vi "test RT Config - Dual RT Sweep.vi"(8 "error in (no error)":errorcluster, 11 "RT Config in":refnum<class "RT Config.lvclass">) -> (0 "error out":errorcluster, 3 "RT Config out":refnum<class "RT Config.lvclass">)   [LabVIEW 2016, in "RT Config.lvclass"]
uses:
  RT Config.lvclass
  Remote Terminal/TypeDefs/RT Configuration.ctl
  Remote Terminal/Remote Terminal.lvclass
  1553 Board/1553 Board.lvclass
  1553 Component/1553 Component.lvclass
  1553 SubComponent/TypeDefs/Scaling Information.ctl
  1553 SubComponent/1553 SubComponent.lvclass
  1553 SubComponent/TypeDefs/Parameter Table Data.ctl
  Remote Terminal/TypeDefs/Command Type.ctl
  Remote Terminal/TypeDefs/Command Configuration.ctl
  D:/SVN/Products/BCI-1553/Software/Development/2016/RealTime/1553 SubComponent/1553 SubComponent.lvclass
  PPLs/FPGA Interface.lvlibp/FPGA Interface/FPGA Interface.lvclass
  Utilities/FPGA Interface/FPGA Interface.lvclass
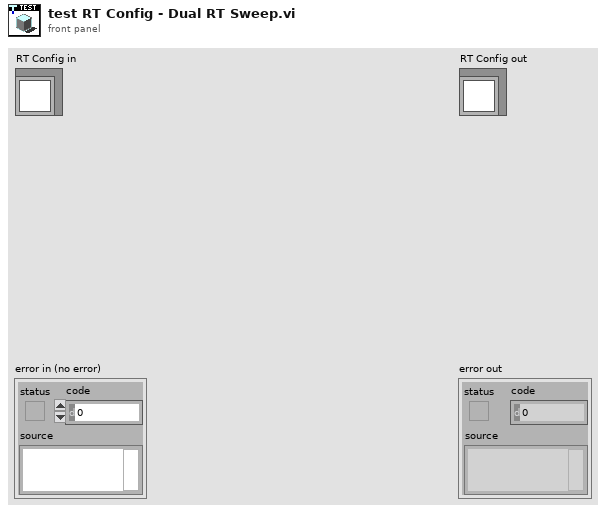
[diagram p1: front panel]
types:
  T1 = typedef "BCI-1553 API.lvlib/Remote Terminal.lvclass/RT Configuration.ctl" = cluster{"RT-RT TimeOut (us)":u8, "Inhibit Bus A":bool, "Inhibit Bus B":bool, "Broadcast CMD Invalid":bool, "UnDef MCs Invalid":bool, "Notice 2 Data Storage":bool, "SMCP":bool, "Temp RX Buffer":bool, "Alt BIT Enable":bool, "Auto Bus Shutdown":bool, "MC 17 Sync":u8, "MC 16 SR Reset":bool, "MC 8 Reset":bool}
  T2 = typedef "BCI-1553 API.lvlib/Remote Terminal.lvclass/Command Type.ctl" = enum16{"Transmit", "Receive", "Mode Code Tx", "Mode Code Rx"}
  T3 = typedef "BCI-1553 API.lvlib/Remote Terminal.lvclass/Command Configuration.ctl" = cluster{"Command Type":T2, "Mode Code ID (1-32)":u16, "SubAddress (1-30)":u16, "Word Count (1-32)":u16, "Illegal Command":bool, "Broadcast":bool, "Data":u16[], "Data Fields":T4[]}
  T4 = typedef "BCI-1553 API.lvlib/1553 SubComponent.lvclass/Parameter Table Data.ctl" = cluster{"Parameter Name":string, "Base Word":u16, "Address":u16, "Value":u64, "Mask":u16[], "Scaling Info":T5}
  T5 = typedef "BCI-1553 API.lvlib/1553 SubComponent.lvclass/Scaling Information.ctl" = cluster{"Bit Offset":i32, "Bit Count":i32, "LSB Resolution":dbl, "2's Complement":bool, "Big Endian":bool, "Sign Bit":bool}
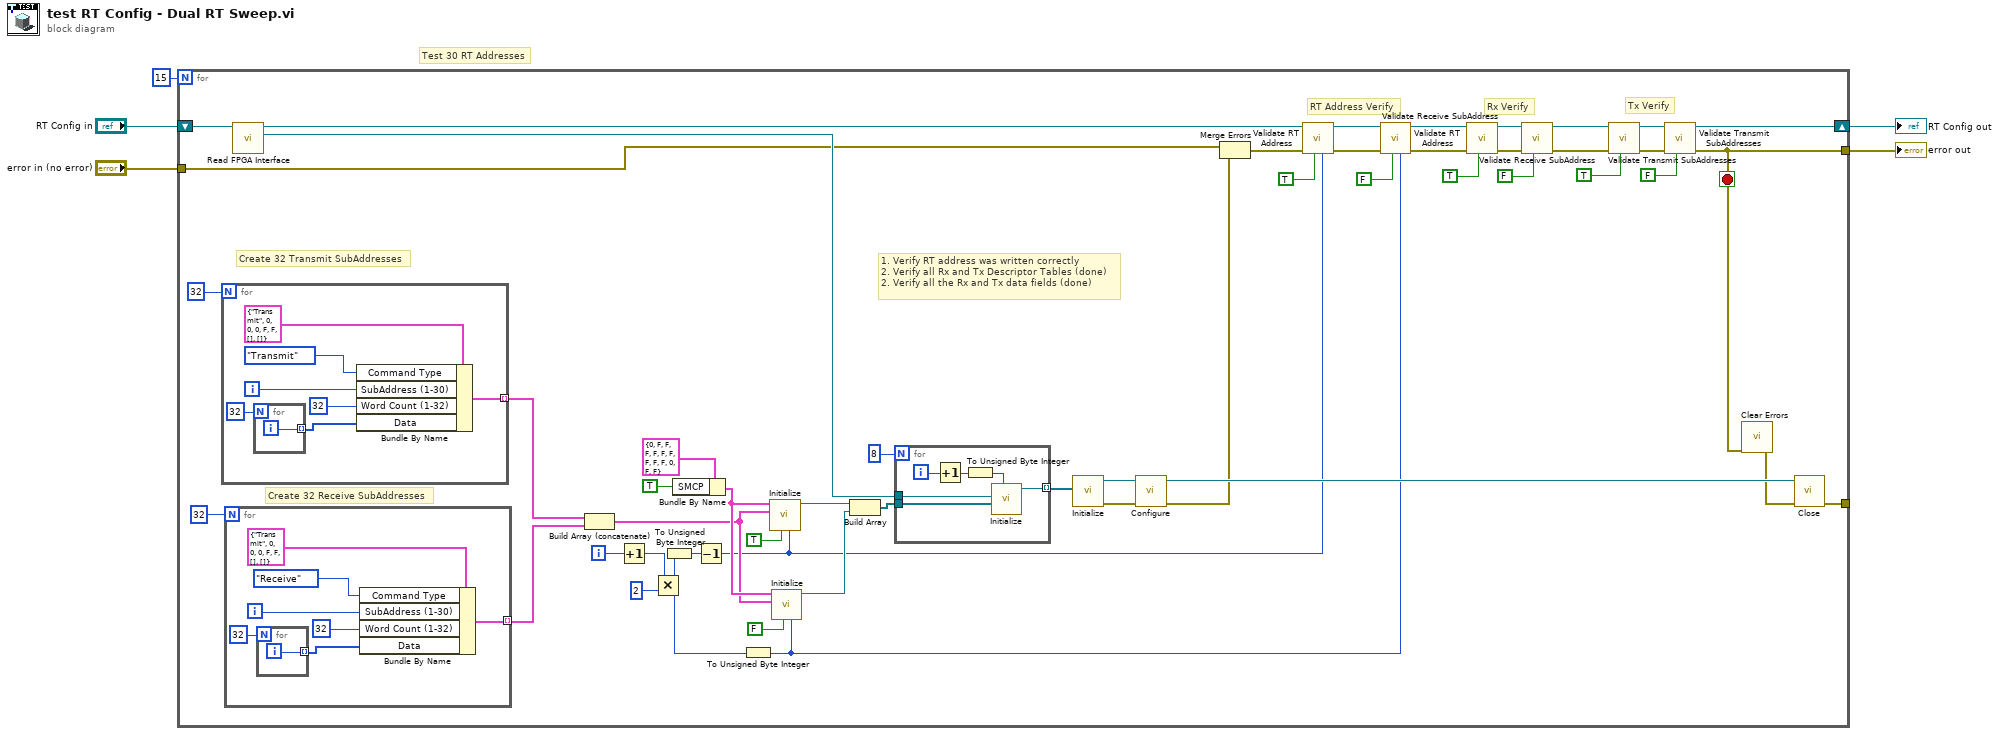
[diagram p0: block diagram]
diagram:
  # "Test 30 RT Addresses"
  n1 = for {
    N: 15 -> [_]
    shift-right: [w9] -> w1
    shift-left: "RT Config in" -> [w45]
    tunnel: [w43] -> _
    tunnel: "error in (no error)" -> [w36]
    tunnel: [w7] -> w2
    i -> [w46]
    stop <- w7 stop-if-true
    # "RT Address Verify"
    # "Rx Verify"
    # "Tx Verify"
    # "1. Verify RT address was written correctly\n2. Verify all Rx and Tx Descriptor Tables (done)\n2. Verify all the Rx and Tx data fields (done)"
    # "Create 32 Receive SubAddresses"
    # "Create 32 Transmit SubAddresses"
    n2 = for {
      N: 32 -> [_]
      tunnel: [w66] -> w39 mode=indexing
      i -> [w65]
      n3 = for {
        N: 32 -> [_]
        tunnel: [w72] -> w67 mode=indexing
        i -> [w72]
      }
      n4 = Bundle By Name(cluster=T3 {"Command Type"=enum."Transmit", "Mode Code ID (1-32)"=0, "SubAddress (1-30)"=0, "Word Count (1-32)"=0, "Illegal Command"=FALSE, "Broadcast"=FALSE, "Data"=[], "Data Fields"=[]} ("CMD Configuration"), "Command Type"=Command_Type."Transmit", "SubAddress (1-30)"=w65, "Word Count (1-32)"=u16 32, "Data"=w67) -> (w66:T3)
    }
    n5 = for {
      N: 32 -> [_]
      tunnel: [w58] -> w40 mode=indexing
      i -> [w57]
      n6 = for {
        N: 32 -> [_]
        tunnel: [w64] -> w59 mode=indexing
        i -> [w64]
      }
      n7 = Bundle By Name(cluster=T3 {"Command Type"=enum."Transmit", "Mode Code ID (1-32)"=0, "SubAddress (1-30)"=0, "Word Count (1-32)"=0, "Illegal Command"=FALSE, "Broadcast"=FALSE, "Data"=[], "Data Fields"=[]} ("CMD Configuration"), "Command Type"=Command_Type."Receive", "SubAddress (1-30)"=w57, "Word Count (1-32)"=u16 32, "Data"=w59) -> (w58:T3)
    }
    n8 = call-dynamic "Read FPGA Interface.vi"("1553 Test in"=w45) -> ("FPGA Interface"=w52:refnum<class "FPGA Interface.lvclass">, "1553 Test out"=w33:refnum<class "RT Config.lvclass">)  [unwired: 8 in, 1 out]
    n9 = Build Array (concatenate)(w39, w40) -> (w29:T3[])
    n10 = Increment(x=w46) -> (x+1=w26:i32)
    n11 = Multiply(x=w26, y=2) -> (x*y=w16:i32)
    n12 = To Unsigned Byte Integer(number=w16) -> (unsigned 8bit integer=w18:u8)
    n13 = Bundle By Name(cluster=T1 {"RT-RT TimeOut (us)"=0, "Inhibit Bus A"=FALSE, "Inhibit Bus B"=FALSE, "Broadcast CMD Invalid"=FALSE, "UnDef MCs Invalid"=FALSE, "Notice 2 Data Storage"=FALSE, "SMCP"=FALSE, "Temp RX Buffer"=FALSE, "Alt BIT Enable"=FALSE, "Auto Bus Shutdown"=FALSE, "MC 17 Sync"=0, "MC 16 SR Reset"=FALSE, "MC 8 Reset"=FALSE} ("RT Configuration"), "SMCP"=TRUE) -> (w30:T1)
    n14 = Decrement(x=w18) -> (x-1=w17:u8)
    n15 = To Unsigned Byte Integer(number=w16) -> (unsigned 8bit integer=w19:u8)
    n16 = call "Initialize.vi"("RT Address (0-30)"=w17, "RT 1?"=TRUE, "Commands"=w29, "RT Configuration"=w30) -> ("Remote Terminal out"=w54:refnum<class "Remote Terminal.lvclass">)  [unwired: 6 in, 1 out]
    n17 = call "Initialize.vi"("RT Address (0-30)"=w19, "RT 1?"=FALSE, "Commands"=w29, "RT Configuration"=w30) -> ("Remote Terminal out"=w25:refnum<class "Remote Terminal.lvclass">)  [unwired: 6 in, 1 out]
    n18 = Build Array(w54, w25) -> (w53:refnum<class "Remote Terminal.lvclass">[])
    n19 = for {
      N: 8 -> [_]
      tunnel: [w76] -> w56 mode=indexing
      tunnel: w53 -> [w75]
      tunnel: w52 -> [w74]
      i -> [w78]
      n20 = Increment(x=w78) -> (x+1=w73:i32)
      n21 = To Unsigned Byte Integer(number=w73) -> (unsigned 8bit integer=w77:u8)
      n22 = call "Initialize.vi"("Component ID (1-8)"=w77, "SubComponents"=w75, "FPGA Interface"=w74) -> ("1553 Component out"=w76:refnum<class "1553 Component.lvclass">)  [unwired: 7 in, 1 out]
    }
    n23 = call "Initialize.vi"("Components"=w56) -> ("error out"=w47:errorcluster, "1553 Board out"=w48:refnum<class "1553 Board.lvclass">)  [unwired: 9 in]
    n24 = call-dynamic "Configure.vi"("error in (no error)"=w47, "1553 Board in"=w48) -> ("error out"=w35:errorcluster, "1553 Board out"=w44:refnum<class "1553 Board.lvclass">)  [unwired: 8 in]
    n25 = Merge Errors(w36, w35) -> (w32:errorcluster)
    n26 = call "Validate RT Address.vi"("RT Address (0-30)"=w17, "RT 1?"=TRUE, "error in (no error)"=w32, "RT Config in"=w33) -> ("error out"=w22:errorcluster, "RT Config out"=w24:refnum<class "RT Config.lvclass">)  [unwired: 6 in]
    n27 = call "Validate RT Address.vi"("RT Address (0-30)"=w19, "RT 1?"=FALSE, "error in (no error)"=w22, "RT Config in"=w24) -> ("error out"=w21:errorcluster, "RT Config out"=w23:refnum<class "RT Config.lvclass">)  [unwired: 6 in]
    n28 = call "Validate Receive SubAddress.vi"("RT 1?"=TRUE, "error in (no error)"=w21, "RT Config in"=w23) -> ("error out"=w13:errorcluster, "RT Config out"=w15:refnum<class "RT Config.lvclass">)  [unwired: 7 in]
    n29 = call "Validate Receive SubAddress.vi"("RT 1?"=FALSE, "error in (no error)"=w13, "RT Config in"=w15) -> ("error out"=w12:errorcluster, "RT Config out"=w14:refnum<class "RT Config.lvclass">)  [unwired: 7 in]
    n30 = call "Validate Transmit SubAddresses.vi"("RT 1?"=TRUE, "error in (no error)"=w12, "RT Config in"=w14) -> ("error out"=w8:errorcluster, "RT Config out"=w10:refnum<class "RT Config.lvclass">)  [unwired: 7 in]
    n31 = call "Validate Transmit SubAddresses.vi"("RT 1?"=FALSE, "error in (no error)"=w8, "RT Config in"=w10) -> ("error out"=w7:errorcluster, "RT Config out"=w9:refnum<class "RT Config.lvclass">)  [unwired: 7 in]
    n32 = call <vilib>:"Clear Errors.vi"("error in (no error)"=w7) -> ("error out"=w37:errorcluster)  [unwired: 5 in, 1 out]
    n33 = call-dynamic "Close.vi"("error in (no error)"=w37, "1553 Board in"=w44) -> ("error out"=w43:errorcluster)  [unwired: 9 in]
  }
  "error out" <- w2
  "RT Config out" <- w1
